vi "Load STL Geometry.vi"(8 "error in (no error)":errorcluster, 11 "Model File":path) -> (0 "error out":errorcluster, 3 "New Mesh Refnum":refnum<vi>)   [LabVIEW 2017, in "NI_3D Picture Control.lvlib"]
doc: "Loads a three-dimensional object model saved in ASCII stereolithography (STL) format to display in a 3D scene."
uses:
  <vilib>/picture/3D Picture Control/NI_3D Picture Control.lvlib
  <vilib>/picture/3D Picture Control/NI_Old 3D Toolkit.lvlib
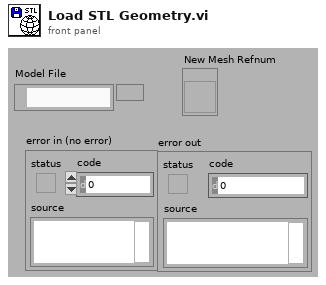
[diagram p1: front panel]
types:
  T1 = typedef "NI_3D Picture Control.lvlib/NI_Old 3D Toolkit.lvlib/model.ctl" = cluster{"VertexList":T2[], "FaceList":cluster{"v1":i32, "v2":i32, "v3":i32}[], "NormalList":T2[], "Mode":T3}
  T2 = typedef "NI_3D Picture Control.lvlib/NI_Old 3D Toolkit.lvlib/point3f.ctl" = cluster{"x":sgl, "y":sgl, "z":sgl}
  T3 = typedef "NI_3D Picture Control.lvlib/NI_Old 3D Toolkit.lvlib/VertexMode.ctl" = enum16{"GL_POINTS", "GL_LINES", "GL_LINE_LOOP", "GL_LINE_STRIP", "GL_TRIANGLES", "GL_TRIANGLE_STRIP", "GL_TRIANGLE_FAN", "GL_QUADS", "GL_QUAD_STRIP", "GL_POLYGON"}
  T4 = enum16{"Points", "Lines", "Line Strip", "Line Loop", "Triangles", "Triangle Strip", "Triangle Fan", "Quads", "Quad Strip", "Polygon"}
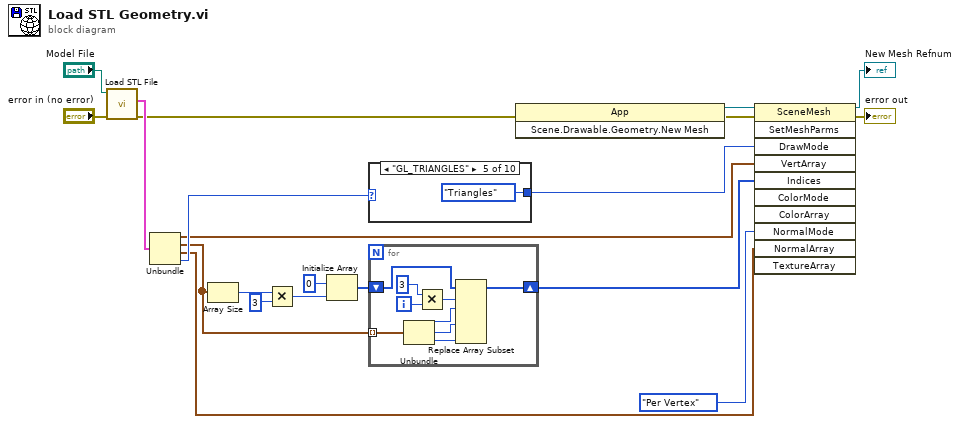
[diagram p0: block diagram]
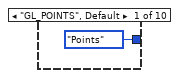
[diagram p2: hidden frame]
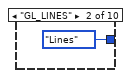
[diagram p3: hidden frame]
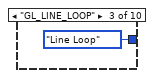
[diagram p4: hidden frame]
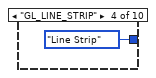
[diagram p5: hidden frame]
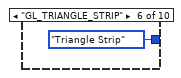
[diagram p6: hidden frame]
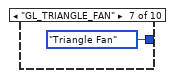
[diagram p7: hidden frame]
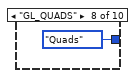
[diagram p8: hidden frame]
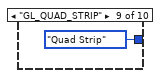
[diagram p9: hidden frame]
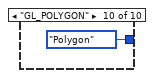
[diagram p10: hidden frame]
diagram:
  n1 = call <vilib>:"Load STL File.vi"("error in (no error)"="error in (no error)", "path to STL file"="Model File") -> ("error out"=w15:errorcluster, "Model Out"=w20:T1)  [unwired: 8 out]
  n2 = Unbundle(w20) -> ("VertexList"=w11:T2[], "FaceList"=w6:cluster{"v1":i32, "v2":i32, "v3":i32}[], "NormalList"=w10:T2[], "Mode"=w19:T3)
  n3 = Array Size(array=w6) -> (size(s)=w2:i32)
  n4 = Multiply(x=w2, y=3 ("x")) -> (x*y=w1:i32)
  n5 = Initialize Array(0 ("v3"), w1) -> (w5:i32[])
  n6 = case shown="\"GL_TRIANGLES\"" w19 {
    tunnel: [T4."Points" ("Draw Mode") T4."Lines" ("Draw Mode") T4."Line Loop" ("Draw Mode") T4."Line Strip" ("Draw Mode") T4."Triangles" ("Draw Mode") T4."Triangle Strip" ("Draw Mode") T4."Triangle Fan" ("Draw Mode") T4."Quads" ("Draw Mode") T4."Quad Strip" ("Draw Mode") T4."Polygon" ("Draw Mode")] -> w7
    frame "GL_POINTS", Default {
    }
    frame "GL_LINES" {
    }
    frame "GL_LINE_LOOP" {
    }
    frame "GL_LINE_STRIP" {
    }
    frame "GL_TRIANGLES" {
    }
    frame "GL_TRIANGLE_STRIP" {
    }
    frame "GL_TRIANGLE_FAN" {
    }
    frame "GL_QUADS" {
    }
    frame "GL_QUAD_STRIP" {
    }
    frame "GL_POLYGON" {
    }
  }
  n7 = for {
    tunnel: w6 -> [w39] mode=indexing
    shift-right: [w38] -> w8
    shift-left: w5 -> [w37]
    i -> [w33]
    n8 = Unbundle(w39) -> ("v1"=w36:i32, "v2"=w35:i32, "v3"=w34:i32)
    n9 = Multiply(x=3, y=w33) -> (x*y=w31:i32)
    n10 = Replace Array Subset(array=w37, new element #1=w36, index #1=w31, new element #2=w35, new element #3=w34) -> (w38:i32[])  [unwired: 2 in]
  }
  n11 = invoke class="App" method="Scene.Drawable.Geometry.New Mesh"(error in=w15) -> (error out=w14:errorcluster, "Scene.Geometry.New Mesh"=w18:refnum<vi>)  [unwired: 2 in, 1 out]
  n12 = invoke class="SceneMesh" method="SetMeshParms"(reference=w18, error in=w14, "DrawMode"=w7, "VertArray"=w11, "Indices"=w8, "NormalMode"=enum16{"Overall", "Per Primitive", "Per Vertex"}."Per Vertex" ("Normal Binding Mode"), "NormalArray"=w10) -> (reference out=→"New Mesh Refnum":refnum<vi>, error out=→"error out":errorcluster)  [unwired: 4 in, 9 out]
